vi "Origin_Z.vi"(0 "PortNumber Z":u8=1) -> (1 "Received String1":string, 2 "Received String2":string="R\r\n", 3 "OK Done":bool)   [LabVIEW 2015]
panel:
  # "Port Number 0=COM1"
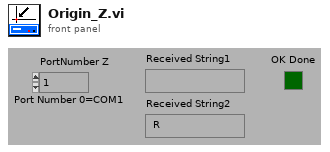
[diagram p1: front panel]
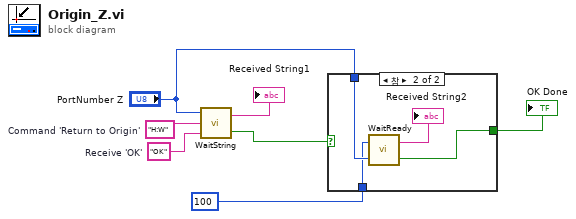
[diagram p0: block diagram]
diagram:
  w4 = "OK"  # Receive 'OK'
  w5 = "H:W"  # Command 'Return to Origin'
  n1 = call "WaitString.vi"("String to Receive"=w4, "String to Send"=w5, "PortNumber"="PortNumber Z") -> ("OK Done"=w2:bool, "String Received"=→"Received String1":string)
  n2 = case shown="참" w2 {
    selector: w2 -> [w8 _]
    tunnel: "PortNumber Z" -> [_ w12]
    tunnel: [w8 w10] -> w7
    tunnel: 100 -> [_ w9]
    frame False {
    }
    frame True {
      n3 = call "WaitReady.vi"("PortNumber"=w12, "Residence time in ms"=w9) -> ("OK Done"=w10:bool, "String Received"=→"Received String2":string)
    }
  }
  "OK Done" <- w7
